vi "waveform to excel_0.vi"() -> ()   [LabVIEW 2015]
uses:
  <vilib>/measure/NI_MABase.lvlib
panel:
  in  "Tab Control":enum32{"Page 1", "Page 2"}(tab)
  out "Waveform Graph":waveform(dbl)(graph)
  in  "stop":bool
  in  "amplitude":dbl=1.0 format="%0.2p"
  in  "frequency":dbl=10.0 format="%0.2p"
  in  "signal type":T1(ring)
  # "Waveform to excel"
  # "Pardeep Kumar"
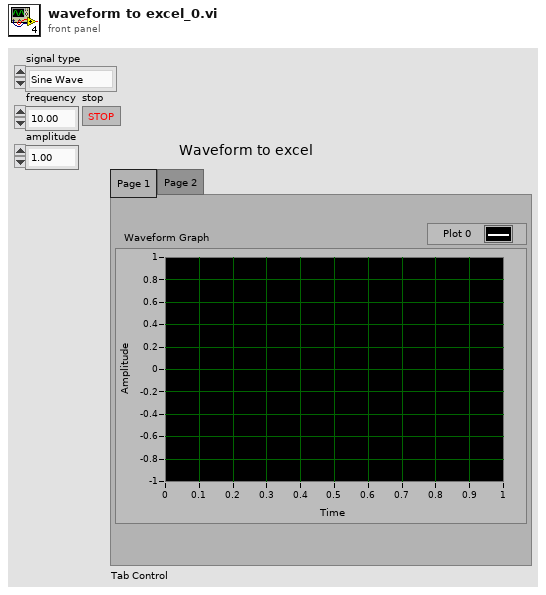
[diagram p1: front panel]
types:
  T1 = enum16{"Sine Wave", "Triangle Wave", "Square Wave", "Sawtooth Wave"}
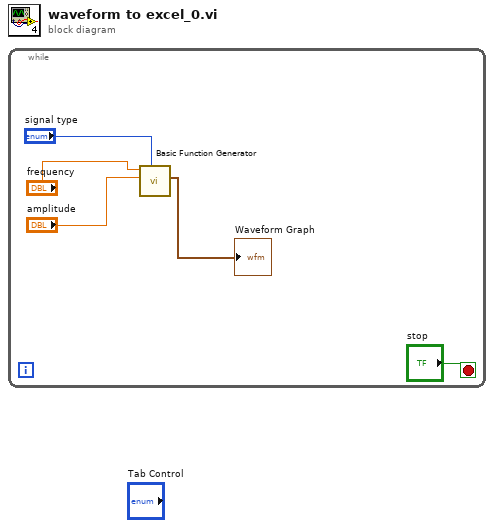
[diagram p0: block diagram]
diagram:
  n1 = while {
    stop <- "stop" stop-if-true
    n2 = call <vilib>:"Basic Function Generator.vi"("signal type"="signal type", "amplitude"="amplitude", "frequency"="frequency") -> ("signal out"=→"Waveform Graph":waveform(dbl))  [unwired: 6 in, 2 out]
  }
